vi "LVClient2011.vi"() -> ()   [LabVIEW 2011]
panel:
  in  "Stop Server":bool
  in  "Stop Client":bool
  in  "Init Button":bool
  in  "Play Button":bool
  out "Python server reply (9 bytes)":string
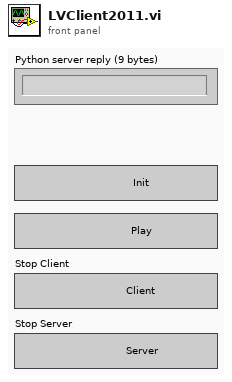
[diagram p1: front panel]
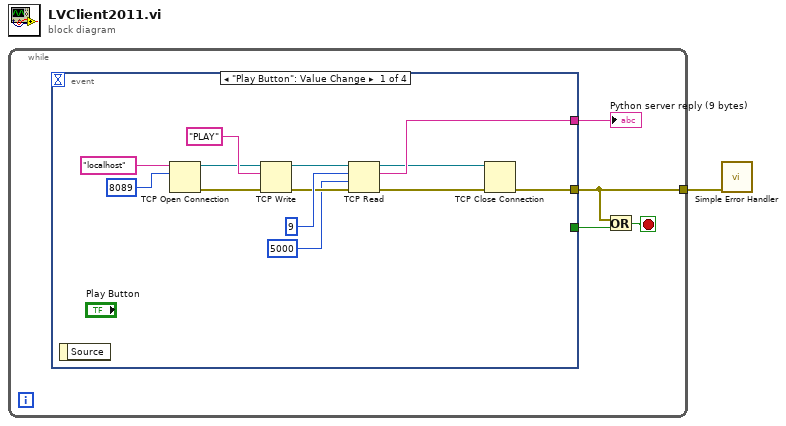
[diagram p0: block diagram]
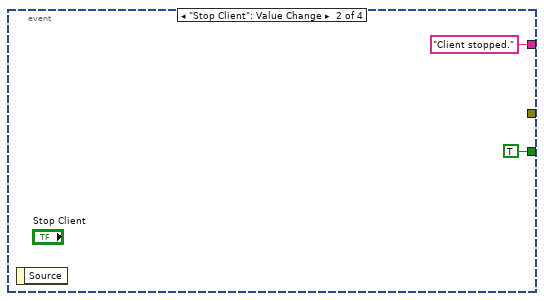
[diagram p2: hidden frame]
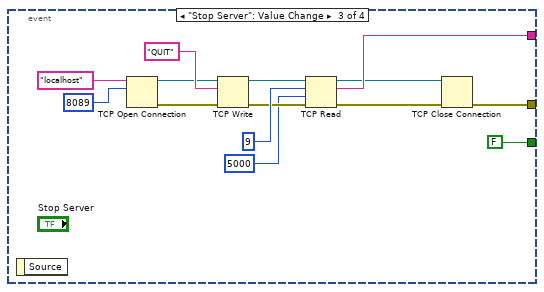
[diagram p3: hidden frame]
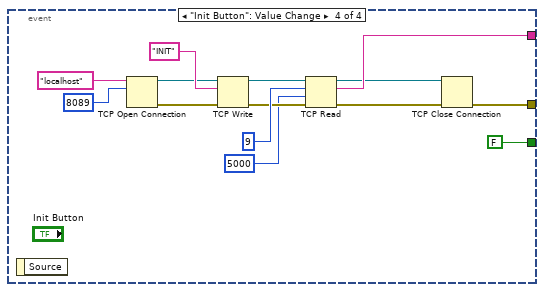
[diagram p4: hidden frame]
diagram:
  n1 = while {
    tunnel: [w4] -> w1
    stop <- w3 stop-if-true
    n2 = event shown="[0] \"Play Button\": Value Change" {
      selector: _ -> [_ _ _ _]
      dyn-events: _ -> [_ _ _ _]
      timeout: _ -> [_ _ _ _]
      tunnel: [w6 _ w22 w36] -> w4
      tunnel: [w13 "Client stopped." ("data out") w29 w43] -> w5
      tunnel: [_ TRUE FALSE FALSE] -> w2
      event "Play Button": Value Change {
        n3 = event-data() -> ()  [unwired: 1 in, 1 out]
        n4 = TCP Open Connection(address="localhost", remote port or service name=u16 8089) -> (connection ID=w10:refnum<k5>, error out=w9:errorcluster)  [unwired: 3 in]
        n5 = TCP Write(connection ID=w10, data in="PLAY", error in (no error)=w9) -> (connection ID out=w16:refnum<k5>, error out=w15:errorcluster)  [unwired: 1 in, 1 out]
        n6 = TCP Read(connection ID=w16, bytes to read=9, error in (no error)=w15, 9:5000 ("timeout ms (25000)")) -> (connection ID out=w8:refnum<k5>, data out=w13:string, error out=w7:errorcluster)  [unwired: 1 in]
        n7 = TCP Close Connection(connection ID=w8, error in (no error)=w7) -> (error out=w6:errorcluster)  [unwired: 1 in, 1 out]
      }
      event "Stop Client": Value Change {
        n8 = event-data() -> ()  [unwired: 1 in, 1 out]
      }
      event "Stop Server": Value Change {
        n9 = event-data() -> ()  [unwired: 1 in, 1 out]
        n10 = TCP Open Connection(address="localhost", remote port or service name=u16 8089) -> (connection ID=w26:refnum<k5>, error out=w25:errorcluster)  [unwired: 3 in]
        n11 = TCP Write(connection ID=w26, data in="QUIT", error in (no error)=w25) -> (connection ID out=w32:refnum<k5>, error out=w31:errorcluster)  [unwired: 1 in, 1 out]
        n12 = TCP Read(connection ID=w32, bytes to read=9, error in (no error)=w31, 9:5000 ("timeout ms (25000)")) -> (connection ID out=w24:refnum<k5>, data out=w29:string, error out=w23:errorcluster)  [unwired: 1 in]
        n13 = TCP Close Connection(connection ID=w24, error in (no error)=w23) -> (error out=w22:errorcluster)  [unwired: 1 in, 1 out]
      }
      event "Init Button": Value Change {
        n14 = event-data() -> ()  [unwired: 1 in, 1 out]
        n15 = TCP Open Connection(address="localhost", remote port or service name=u16 8089) -> (connection ID=w40:refnum<k5>, error out=w39:errorcluster)  [unwired: 3 in]
        n16 = TCP Write(connection ID=w40, data in="INIT", error in (no error)=w39) -> (connection ID out=w46:refnum<k5>, error out=w45:errorcluster)  [unwired: 1 in, 1 out]
        n17 = TCP Read(connection ID=w46, bytes to read=9, error in (no error)=w45, 9:5000 ("timeout ms (25000)")) -> (connection ID out=w38:refnum<k5>, data out=w43:string, error out=w37:errorcluster)  [unwired: 1 in]
        n18 = TCP Close Connection(connection ID=w38, error in (no error)=w37) -> (error out=w36:errorcluster)  [unwired: 1 in, 1 out]
      }
    }
    "Python server reply (9 bytes)" <- w5
    n19 = Or(x=w4, y=w2) -> (x .or. y?=w3:bool)
  }
  n20 = call <vilib>:"Simple Error Handler.vi"("error in (no error)"=w1) -> ()  [unwired: 4 in, 5 out]
